vi "Manage DataPlugins.vi"(8 "error in (no error)":errorcluster) -> (0 "error out":errorcluster)   [LabVIEW 2020]
doc: "This example demonstrates how to use the Manage DataPlugins VIs to create a DataPlugin Manager application. The DataPlugin Manager application lists all DataPlugins, including the name, type, file extensions, and version information, installed on the local computer when you first open this application. You can use this application to import, export, encrypt, or remove DataPlugins. \n\nImporting a DataPlugin registers the DataPlugin to the local computer. After you download a DataPlugin .uri file from the National Instruments Web site at ni.com/dataplugins, click the <B>Import</B> button to import the DataPlugin to the DataPlugin Manager. You then can use the DataPlugin to access the corresponding file format.\n\nExporting a DataPlugin enables you to generate a DataPlugin .uri file from a DataPlugin that you created in NI DIAdem. After you create a DataPlugin, the name and related information appears in the DataPlugin Manager. Select the DataPlugin and click the <B>Export</B> button to export the DataPlugin to a .uri file. You then can distribute the .uri file to other users. To export an encrypted DataPlugin, click the <B>Encrypt</B> button. Refer to ni.com/diadem for more information about NI DIAdem.\n\n\nRemoving a DataPlugin unregisters the DataPlugin from the local computer. Select the DataPlugin you want to remove and click the <B>Remove</B> button. This button does not delete the corresponding DataPlugin .uri file or installer from the computer.\n\n<B>Note:</B> DataPlugins are shared between different National Instruments products and applications on the local computer. Registering or unregistering a DataPlugin might affect these products or applications.\n\nClick the <B>Close</B> button the exit the run mode of this application. Open the block diagram of this application for more information about using the DataPlugin Manager VIs."
uses:
  <vilib>/Platform/storage/utility/Register DataPlugin by URI.vi
panel:
  in  "encrypt":bool
  in  "remove":bool
  in  "export":bool
  in  "close":bool
  in  "import":bool
  in  "DataPlugin Settings":i32(listbox)
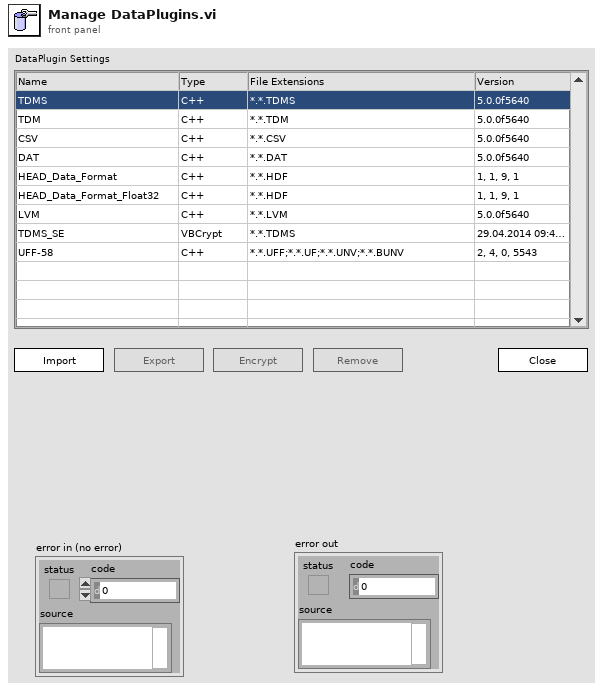
[diagram p1: front panel]
types:
  T1 = enum8{"Enabled", "Disabled", "Disabled and Grayed Out"}
  T2 = typedef "usiPluginInformation.ctl" = cluster{"name":string, "version":string, "type":string, "read-only?":bool, "extensions":string[]}
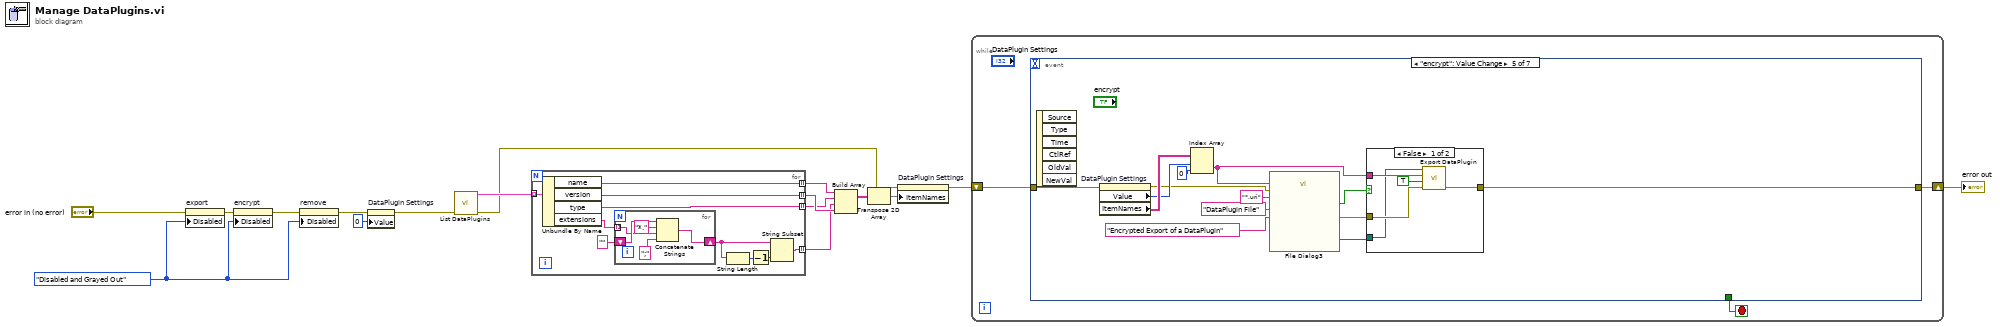
[diagram p0: block diagram]
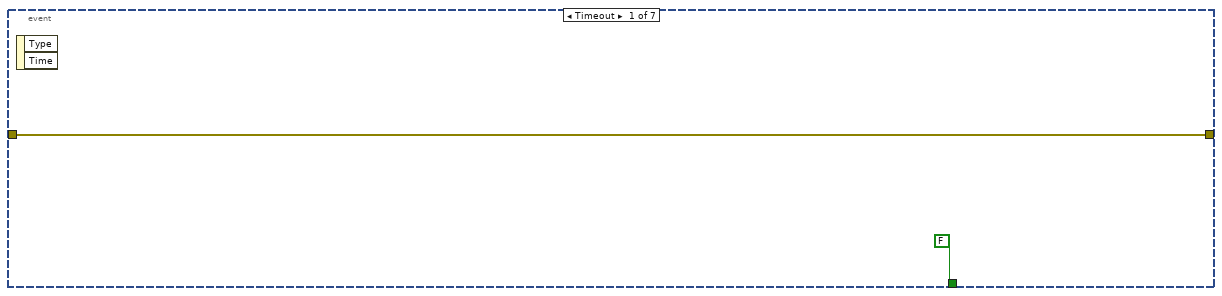
[diagram p2: hidden frame]
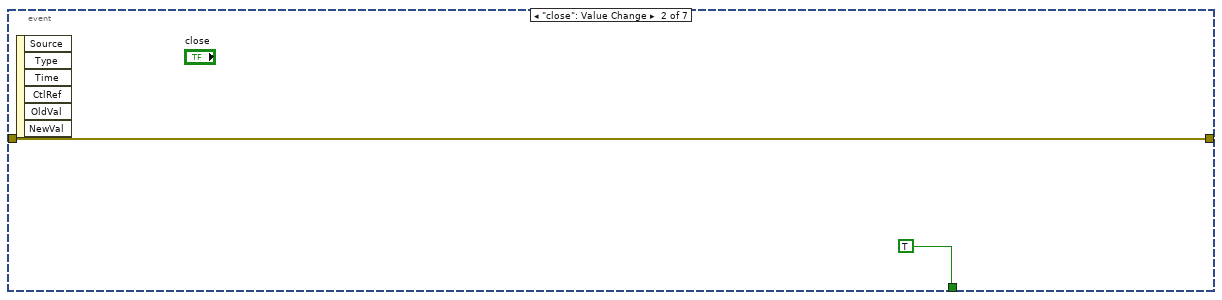
[diagram p3: hidden frame]
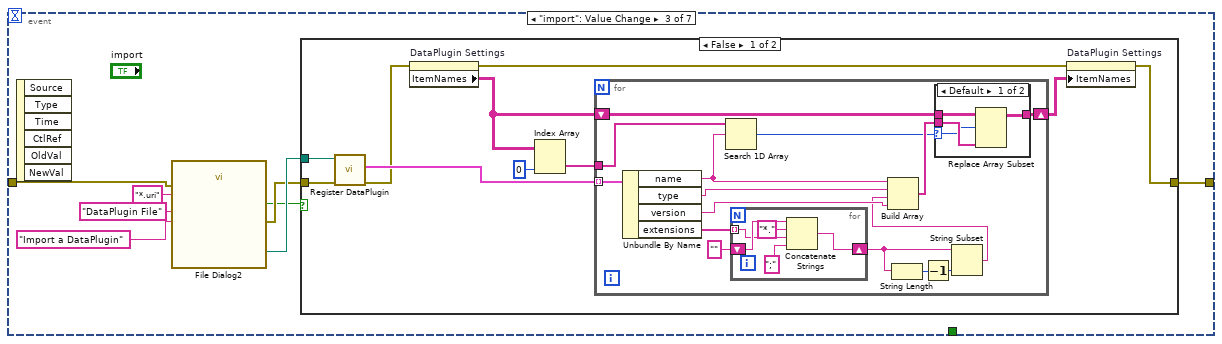
[diagram p4: hidden frame]
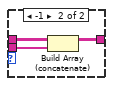
[diagram p5: hidden frame]
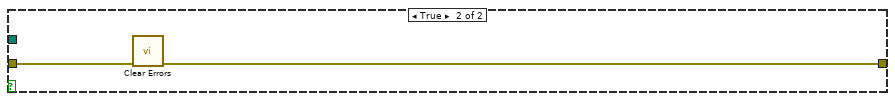
[diagram p6: hidden frame]
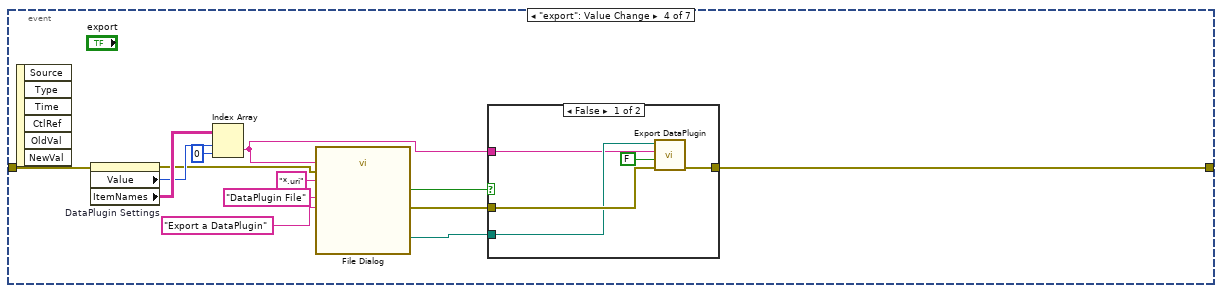
[diagram p7: hidden frame]
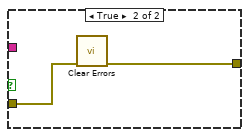
[diagram p8: hidden frame]
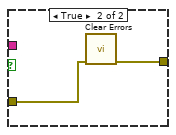
[diagram p9: hidden frame]
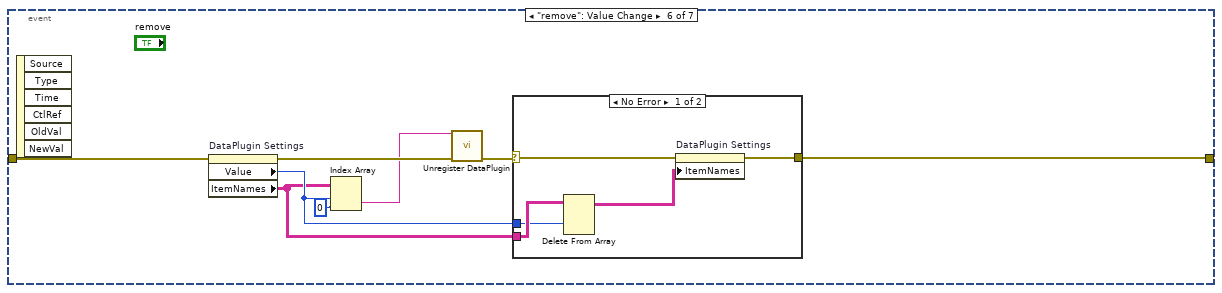
[diagram p10: hidden frame]
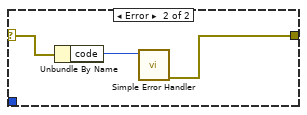
[diagram p11: hidden frame]
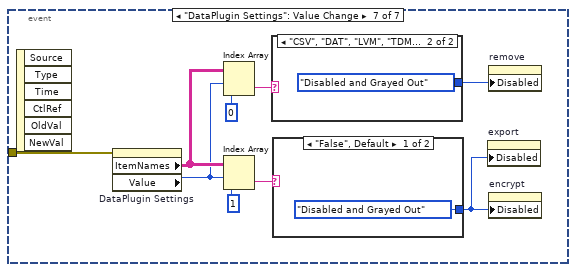
[diagram p12: hidden frame]
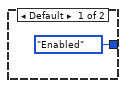
[diagram p13: hidden frame]
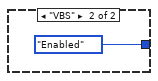
[diagram p14: hidden frame]
diagram:
  w3 = T1."Disabled and Grayed Out" ("Disabled")
  n1 = property on="export" class="Bool"(error in="error in (no error)", "Disabled"=w3) -> (error out=w4:errorcluster)  [unwired: 1 in, 1 out]
  n2 = property on="encrypt" class="Bool"(error in=w4, "Disabled"=w3) -> (error out=w2:errorcluster)  [unwired: 1 in, 1 out]
  n3 = property on="remove" class="Bool"(error in=w2, "Disabled"=w3) -> (error out=w5:errorcluster)  [unwired: 1 in, 1 out]
  n4 = property on="DataPlugin Settings" class="MCListbox (strict)"(error in=w5, "Value"=0 ("DataPlugin Settings")) -> (error out=w11:errorcluster)  [unwired: 1 in, 1 out]
  n5 = call <vilib>:"List DataPlugins.vi"("error in (no error)"=w11) -> ("DataPlugin information"=w13:T2[], "error out"=w12:errorcluster)  [unwired: 13 in]
  n6 = for {
    tunnel: w13 -> [w26] mode=indexing
    tunnel: [w24] -> w14 mode=indexing
    tunnel: [w19] -> w6 mode=indexing
    tunnel: [w23] -> w8 mode=indexing
    tunnel: [w22] -> w7 mode=indexing
    n7 = Unbundle By Name(w26) -> ("name"=w24:string, "version"=w23:string, "type"=w22:string, "extensions"=w25:string[])
    n8 = for {
      tunnel: w25 -> [w29] mode=indexing
      shift-right: [w32] -> w20
      shift-left: "" ("extensions") -> [w31]
      n9 = Concatenate Strings(w31, "*." ("string"), w29, ";" ("string")) -> (w32:string)
    }
    n10 = String Length(string=w20) -> (length=w21:i32)
    n11 = Decrement(x=w21) -> (x-1=w18:i32)
    n12 = String Subset(string=w20, length (rest)=w18) -> (substring=w19:string)  [unwired: 1 in]
  }
  n13 = Build Array(w14, w7, w6, w8) -> (w17:string[][])
  n14 = Transpose 2D Array(2D array=w17) -> (transposed array=w15:string[][])
  n15 = property on="DataPlugin Settings" class="MCListbox (strict)"(error in=w12, "ItemNames"=w15) -> (error out=w9:errorcluster)  [unwired: 1 in, 1 out]
  n16 = while {
    shift-right: [w33] -> w16
    shift-left: w9 -> [w34]
    stop <- w35 stop-if-true
    n17 = event shown="[4] \"encrypt\": Value Change" {
      selector: _ -> [_ _ _ _ _ _ _]
      dyn-events: _ -> [_ _ _ _ _ _ _]
      timeout: _ -> [_ _ _ _ _ _ _]
      tunnel: [FALSE TRUE _ _ _ _ _] -> w35
      tunnel: w34 -> [w36 w38 w44 w89 w109 w133 w151]
      tunnel: [w36 w38 w43 w93 w112 w128 _] -> w33
      event Timeout {
        n18 = event-data() -> ()  [unwired: 3 out]
      }
      event "close": Value Change {
        n19 = event-data() -> ()  [unwired: 7 out]
      }
      event "import": Value Change {
        n20 = event-data() -> ()  [unwired: 7 out]
        n21 = call "File Dialog2"("prompt"="Import a DataPlugin" ("button label"), "error in"=w44, "pattern (all files)"="*.uri", "pattern label"="DataPlugin File") -> ("selected path"=w42:path, "cancelled"=w40:bool, "error out"=w41:errorcluster)  [unwired: 8 in, 1 out]
        n22 = case shown="False" w40 {
          tunnel: [w54 w85] -> w43
          tunnel: w42 -> [w57 _]
          tunnel: w41 -> [w56 w86]
          frame False {
            n23 = call-poly <vilib>:"Register DataPlugin.vi"("error in (no error)"=w56, "DataPlugin URI path (*.uri)"=w57) -> ("error out"=w53:errorcluster, "DataPlugin information"=w55:T2[])  [unwired: 7 in, 1 out]
            n24 = property on="DataPlugin Settings" class="MCListbox (strict)"(error in=w53) -> (error out=w52:errorcluster, "ItemNames"=w49:string[][])  [unwired: 1 in, 1 out]
            n25 = Index Array(array=w49, index (col)=0 ("disabled index (col)")) -> (element=w50:string[])  [unwired: 1 in]
            n26 = for {
              tunnel: w55 -> [w72] mode=indexing
              tunnel: w50 -> [w64]
              shift-right: [w66] -> w48
              shift-left: w49 -> [w65]
              n27 = Unbundle By Name(w72) -> ("name"=w63:string, "type"=w69:string, "version"=w68:string, "extensions"=w71:string[])
              n28 = Search 1D Array(1D array=w64, element=w63) -> (index of element=w62:i32)  [unwired: 1 in]
              n29 = for {
                tunnel: w71 -> [w81] mode=indexing
                shift-right: [w84] -> w59
                shift-left: "" -> [w83]
                n30 = Concatenate Strings(w83, "*." ("string"), w81, ";" ("string")) -> (w84:string)
              }
              n31 = String Length(string=w59) -> (length=w61:i32)
              n32 = Decrement(x=w61) -> (x-1=w60:i32)
              n33 = String Subset(string=w59, length (rest)=w60) -> (substring=w58:string)  [unwired: 1 in]
              n34 = Build Array(w63, w69, w58, w68) -> (w67:string[])
              n35 = case shown="Default" w62 {
                selector: w62 -> [w74 _]
                tunnel: w67 -> [w75 w79]
                tunnel: [w73 w78] -> w66
                tunnel: w65 -> [w76 w77]
                frame Default {
                  n36 = Replace Array Subset(array=w76, new element=w75, index (row)=w74) -> (w73:string[][])  [unwired: 1 in]
                }
                frame -1 {
                  n37 = Build Array (concatenate)(w77, w79) -> (w78:string[][])
                }
              }
            }
            n38 = property on="DataPlugin Settings" class="MCListbox (strict)"(error in=w52, "ItemNames"=w48) -> (error out=w54:errorcluster)  [unwired: 1 in, 1 out]
          }
          frame True {
            n39 = call <vilib>:"Clear Errors.vi"("error in (no error)"=w86) -> ("error out"=w85:errorcluster)  [unwired: 5 in, 1 out]
          }
        }
      }
      event "export": Value Change {
        n40 = event-data() -> ()  [unwired: 7 out]
        n41 = property on="DataPlugin Settings" class="MCListbox (strict)"(error in=w89) -> (error out=w88:errorcluster, "Value"=w95:i32, "ItemNames"=w96:string[][])  [unwired: 1 in, 1 out]
        n42 = Index Array(array=w96, index (row)=w95, index (col)=0 ("disabled index (col)")) -> (element=w90:string)
        n43 = call "File Dialog"("prompt"="Export a DataPlugin" ("button label"), "default name"=w90, "error in"=w88, "pattern (all files)"="*.uri", "pattern label"="DataPlugin File") -> ("selected path"=w91:path, "cancelled"=w87:bool, "error out"=w92:errorcluster)  [unwired: 7 in, 1 out]
        n44 = case shown="False" w87 {
          tunnel: [w103 w105] -> w93
          tunnel: w92 -> [w102 w106]
          tunnel: w91 -> [w101 _]
          tunnel: w90 -> [w100 _]
          frame False {
            n45 = call <vilib>:"Export DataPlugin.vi"("error in (no error)"=w102, "encrypt? (F)"=FALSE ("encrypted? (no)"), "DataPlugin name"=w100, "DataPlugin URI path (*.uri)"=w101) -> ("error out"=w103:errorcluster)  [unwired: 6 in, 1 out]
          }
          frame True {
            n46 = call <vilib>:"Clear Errors.vi"("error in (no error)"=w106) -> ("error out"=w105:errorcluster)  [unwired: 5 in, 1 out]
          }
        }
      }
      event "encrypt": Value Change {
        n47 = event-data() -> ()  [unwired: 7 out]
        n48 = property on="DataPlugin Settings" class="MCListbox (strict)"(error in=w109) -> (error out=w108:errorcluster, "Value"=w115:i32, "ItemNames"=w116:string[][])  [unwired: 1 in, 1 out]
        n49 = Index Array(array=w116, index (row)=w115, index (col)=0 ("disabled index (col)")) -> (element=w111:string)
        n50 = call "File Dialog3"("prompt"="Encrypted Export of a DataPlugin" ("button label"), "default name"=w111, "error in"=w108, "pattern (all files)"="*.uri", "pattern label"="DataPlugin File") -> ("selected path"=w110:path, "cancelled"=w107:bool, "error out"=w113:errorcluster)  [unwired: 7 in, 1 out]
        n51 = case shown="False" w107 {
          tunnel: w113 -> [w124 w126]
          tunnel: [w123 w125] -> w112
          tunnel: w111 -> [w122 _]
          tunnel: w110 -> [w121 _]
          frame False {
            n52 = call <vilib>:"Export DataPlugin.vi"("error in (no error)"=w124, "encrypt? (F)"=TRUE ("encrypted? (no)"), "DataPlugin name"=w122, "DataPlugin URI path (*.uri)"=w121) -> ("error out"=w123:errorcluster)  [unwired: 6 in, 1 out]
          }
          frame True {
            n53 = call <vilib>:"Clear Errors.vi"("error in (no error)"=w126) -> ("error out"=w125:errorcluster)  [unwired: 5 in, 1 out]
          }
        }
      }
      event "remove": Value Change {
        n54 = event-data() -> ()  [unwired: 7 out]
        n55 = property on="DataPlugin Settings" class="MCListbox (strict)"(error in=w133) -> (error out=w132:errorcluster, "Value"=w129:i32, "ItemNames"=w127:string[][])  [unwired: 1 in, 1 out]
        n56 = Index Array(array=w127, index (row)=w129, index (col)=0 ("disabled index (col)")) -> (element=w131:string)
        n57 = call <vilib>:"Unregister DataPlugin.vi"("DataPlugin name"=w131, "error in (no error)"=w132) -> ("error out"=w130:errorcluster)  [unwired: 13 in]
        n58 = case shown="No Error" w130 {
          selector: w130 -> [w139 w142]
          tunnel: w129 -> [w136 _]
          tunnel: [w138 w140] -> w128
          tunnel: w127 -> [w137 _]
          frame No Error {
            n59 = Delete From Array(array=w137, index (row)=w136) -> (array with subset deleted=w135:string[][])  [unwired: 2 in, 1 out]
            n60 = property on="DataPlugin Settings" class="MCListbox (strict)"(error in=w139, "ItemNames"=w135) -> (error out=w138:errorcluster)  [unwired: 1 in, 1 out]
          }
          frame Error {
            n61 = Unbundle By Name(w142) -> ("code"=w141:i32)
            n62 = call <vilib>:"Simple Error Handler.vi"("error code (no error:0)"=w141) -> ("error out"=w140:errorcluster)  [unwired: 4 in, 4 out]
          }
        }
      }
      event "DataPlugin Settings": Value Change {
        n63 = event-data() -> ()  [unwired: 7 out]
        n64 = property on="DataPlugin Settings" class="MCListbox (strict)"(error in=w151) -> ("ItemNames"=w146:string[][], "Value"=w145:i32)  [unwired: 1 in, 2 out]
        n65 = Index Array(array=w146, index (row)=w145, index (col)=0 ("disabled index (col)")) -> (element=w144:string)
        n66 = Index Array(array=w146, index (row)=w145, index (col)=1 ("disabled index (col)")) -> (element=w149:string)
        n67 = case shown="\"CSV\", \"DAT\", \"LVM\", \"TDM\", \"TDMS\"" w144 {
          tunnel: [T1."Enabled" ("Disabled") T1."Disabled and Grayed Out" ("Disabled")] -> w143
          frame Default {
          }
          frame "CSV", "DAT", "LVM", "TDM", "TDMS" {
          }
        }
        n68 = case shown="\"False\", Default" w149 {
          tunnel: [T1."Disabled and Grayed Out" ("Disabled") T1."Enabled" ("Disabled")] -> w148
          frame "False", Default {
          }
          frame "VBS" {
          }
        }
        n69 = property on="export" class="Bool"("Disabled"=w148) -> ()  [unwired: 2 in, 2 out]
        n70 = property on="remove" class="Bool"("Disabled"=w143) -> ()  [unwired: 2 in, 2 out]
        n71 = property on="encrypt" class="Bool"("Disabled"=w148) -> ()  [unwired: 2 in, 2 out]
      }
    }
  }
  "error out" <- w16
